vi "trig EMCCD.vi"(1 "error in (no error)":errorcluster, 2 "camera time":dbl, 3 "lines":tag="Dev1/port0/line0") -> (0 "error out":errorcluster)   [LabVIEW 2018]
uses:
  <vilib>/DAQmx/write.llb/DAQmx Write (Digital Bool 1Line 1Point).vi
  <vilib>/DAQmx/create/channels.llb/DAQmx Create Channel (DO-Digital Output).vi
  <vilib>/DAQmx/miscellaneous.llb/DAQmx Fill In Error Info.vi
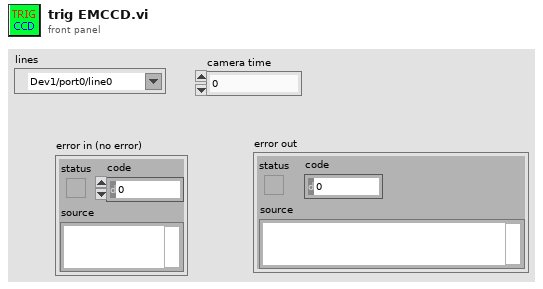
[diagram p1: front panel]
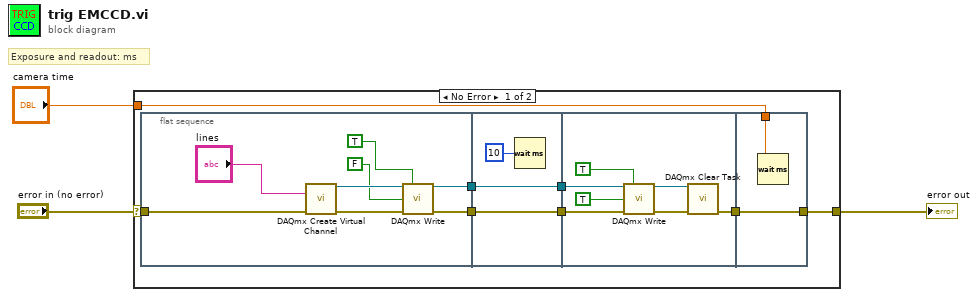
[diagram p0: block diagram]
diagram:
  # "Exposure and readout: ms"
  n1 = case shown="No Error" "error in (no error)" {
    selector: "error in (no error)" -> [w9 w32]
    tunnel: [w6 w32] -> w2
    tunnel: "camera time" -> [w4 _]
    frame No Error {
      n2 = flat-sequence {
        tunnel: [w15] -> w11
        tunnel: [w13] -> w7
        tunnel: w9 -> [w12]
        tunnel: w11 -> [w21]
        tunnel: [w21] -> w10
        tunnel: [w20] -> w8
        tunnel: w7 -> [w20]
        tunnel: w8 -> [w25]
        tunnel: w10 -> [w26]
        tunnel: [w23] -> w5
        tunnel: [w31] -> w6
        tunnel: w5 -> [w31]
        tunnel: w4 -> [w30]
        frame #0 {
          n3 = call-poly <vilib>:"DAQmx Create Virtual Channel.vi"("lines"="lines", "error in"=w12) -> ("task out"=w17:refnum<k21>, "error out"=w14:errorcluster)  [unwired: 12 in]
          n4 = call-poly <vilib>:"DAQmx Write.vi"("task/channels in"=w17, "auto start"=TRUE, "data"=FALSE ("Shutter"), "error in"=w14) -> ("task out"=w15:refnum<k21>, "error out"=w13:errorcluster)  [unwired: 9 in, 1 out]
        }
        frame #1 {
          n5 = Wait (ms)(milliseconds to wait=u32 10) -> ()  [unwired: 1 out]
        }
        frame #2 {
          n6 = call-poly <vilib>:"DAQmx Write.vi"("task/channels in"=w26, "auto start"=TRUE, "data"=TRUE, "error in"=w25) -> ("task out"=w29:refnum<k21>, "error out"=w24:errorcluster)  [unwired: 9 in, 1 out]
          n7 = call <vilib>:"DAQmx Clear Task.vi"("task in"=w29, "error in"=w24) -> ("error out"=w23:errorcluster)  [unwired: 13 in]
        }
        frame #3 {
          n8 = Wait (ms)(milliseconds to wait=w30) -> ()  [unwired: 1 out]
        }
      }
    }
    frame Error {
    }
  }
  "error out" <- w2
